vi "System Set Points and States.vi"() -> ()   [LabVIEW 2012]
uses:
  <vilib>/Rock Robotics/WPI/Joystick/WPI_JoystickButtonState.ctl
panel:
  out "Angle Set Point":dbl
  out "Gyro Angle":dbl
  out "Drive Dist":dbl
  out "Right Distance":dbl
  out "Left Distance":dbl
  out "Left Drive Set":dbl
  out "Right Drive Set":dbl
  out "Right Drive":dbl
  out "Left Drive":dbl
  out "Right Drive JS":dbl
  out "Left Drive JS":dbl
  in  "Shot":bool
  in  "Collect Backward":bool
  in  "Collect Forward":bool
  out "Encoder 1 Distance":dbl
  in  "PID Stable 2":bool
  out "Encoder 2 Distance":dbl
  out "Shooter 2 Set Speed":dbl
  out "Shooter RPM 2":dbl
  out "Open Loop PWM 2":dbl
  out "ShooterDiff":dbl
  in  "PID Stable":bool
  out "CountDown":dbl
  out "Camera Enabled":bool
  out "Axes":T1
  out "Buttons":T2
  out "Shooter RPM":dbl
  out "Open Loop PWM":dbl
  in  "Open Loop":bool
  in  "Shooter Enabled":bool
  out "Shooter Set Speed":dbl
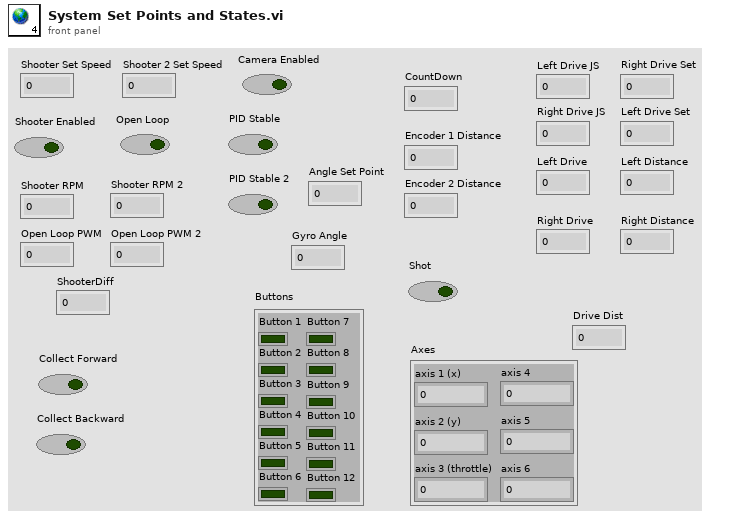
[diagram p1: front panel]
types:
  T1 = cluster{"axis 1 (x)":dbl, "axis 2 (y)":dbl, "axis 3 (throttle)":dbl, "axis 4":dbl, "axis 5":dbl, "axis 6":dbl}
  T2 = typedef "WPI_JoystickButtonState.ctl" = cluster{"Button 1":bool, "Button 2":bool, "Button 3":bool, "Button 4":bool, "Button 5":bool, "Button 6":bool, "Button 7":bool, "Button 8":bool, "Button 9":bool, "Button 10":bool, "Button 11":bool, "Button 12":bool}
diagram:
